vi "Refresh All Pages.vi"() -> ()   [LabVIEW 2014]
uses:
  <vilib>/Platform/browser.llb/Open URL in Default Browser (string).vi
panel:
  in  "Wiki Help Base URL":string="https://www.labviewmakerhub.com/doku.php?id=learn:libraries:linx:reference:labview:"
  out "Array":string[](array[string])=["\\analog-read-1-chan.txt", "\\analog-read-n-chans.txt", "\\analog-set-reference-voltage.txt", "\\analog-write-1-chan.txt", "\\analog-write-n-chans.txt", "\\check-channel.txt", "\\close.txt", "\\custom-command.txt", "\\digital-close.txt", "\\digital-read-1-chan.txt", "\\digital-read-n-chans.txt", "\\digital-read-pulse-width.txt", "\\digital-write-1-chan.txt", "\\digital-write-n-chans.txt", "\\digital-write-square-wave.txt", "\\get-device-user-id.txt", "\\i2c-close.txt", "\\i2c-open.txt", "\\i2c-read.txt", "\\i2c-write.txt", "\\initialize.txt", "\\open-local.txt", "\\open-serial.txt", "\\open-tcp.txt", "\\photocell.txt", "\\pwm-set-duty-cycle-1-chan.txt", "\\pwm-set-duty-cycle-n-chans.txt", "\\rgb-led.txt", "\\set-device-user-id.txt", "\\seven-segment-display.txt", "\\spi-configure.txt", "\\spi-open.txt", "\\spi-write-read-1-frame.txt", "\\spi-write-read-n-frames.txt", "\\thermistor.txt", "\\thumbstick.txt", "\\uart-close.txt", "\\uart-get-bytes-available.txt", "\\uart-open.txt", "\\uart-read-byte-array.txt", "\\uart-read-string.txt", "\\uart-set-baud-rate.txt", "\\uart-write-byte-array.txt", "\\uart-write-string.txt", "\\ad9850\\open.txt", "\\ad9850\\set-frequency-and-phase.txt", "\\adxl345\\close.txt", "\\adxl345\\open.txt", "\\adxl345\\read.txt", "\\blinkm\\go-to-rgb-color-now.txt", "\\blinkm\\open.txt", "\\ds1307\\open.txt", "\\ds1307\\read.txt", "\\ds1307\\write.txt", "\\hitechnic\\accelerometer\\close.txt", "\\hitechnic\\accelerometer\\open.txt", "\\hitechnic\\accelerometer\\read.txt", "\\ltc2631\\open.txt", "\\ltc2631\\write.txt", "\\mma8451\\close.txt", "\\mma8451\\open.txt", "\\mma8451\\read.txt", "\\mma8451\\who-am-i.txt", "\\mma8452\\close.txt", "\\mma8452\\open.txt", "\\mma8452\\read.txt", "\\mpu60x0\\close.txt", "\\mpu60x0\\open.txt", "\\mpu60x0\\read.txt", "\\mpu60x0\\set-clock-source.txt", "\\mpu60x0\\set-fullscale-accel-range.txt", "\\mpu60x0\\set-fullscale-gyro-range.txt", "\\mpu60x0\\set-sleep-enabled.txt", "\\pmodacl\\close.txt", "\\pmodacl\\open.txt", "\\pmodacl\\read.txt", "\\pmodals\\open.txt", "\\pmodals\\read.txt", "\\pmodcmps\\close.txt", "\\pmodcmps\\open.txt", "\\pmodcmps\\read.txt", "\\pmodgyro\\close.txt", "\\pmodgyro\\open.txt", "\\pmodgyro\\read.txt", "\\pmodmic3\\open.txt", "\\pmodmic3\\read.txt", "\\pmodtc1\\open.txt", "\\pmodtc1\\read.txt", "\\servo\\servo-close-n-channels.txt", "\\servo\\servo-close-one-channel.txt", "\\servo\\servo-open-n-channels.txt", "\\servo\\servo-open-one-channel.txt", "\\servo\\servo-set-pulse-width-n-channels.txt", "\\servo\\servo-set-pulse-width-one-channel.txt", "\\ssd1306\\2d-bool-array-to-image-data-helper.txt", "\\ssd1306\\channels-fgv.txt", "\\ssd1306\\digilent-basic-io-shield---oled-config.txt", "\\ssd1306\\digilent-basic-io-shield---oled-draw-bool-array.txt", "\\ssd1306\\enable-charge-pump.txt", "\\ssd1306\\open.txt", "\\ssd1306\\png-to-bool-array.txt", "\\ssd1306\\set-column-address-range.txt", "\\ssd1306\\set-com-hw-config.txt", "\\ssd1306\\set-com-output-scan-direction.txt", "\\ssd1306\\set-display-on-off.txt", "\\ssd1306\\set-page.txt", "\\ssd1306\\set-segment-remap.txt", "\\ssd1306\\write-data.txt", "\\tcn75a\\open.txt", "\\tcn75a\\read.txt", "\\tmp3x\\tmp35.txt", "\\tmp3x\\tmp36.txt", "\\tmp3x\\tmp37.txt", "\\ultrasonic\\gh-311.txt", "\\ultrasonic\\hc-sr04.txt", "\\ultrasonic\\ping.txt", "\\ultrasonic\\read.txt", "\\ws2812\\close.txt", "\\ws2812\\open.txt", "\\ws2812\\refresh.txt", "\\ws2812\\write-n-leds.txt", "\\ws2812\\write-one-led.txt"]
  in  "File Path Control":path=path "C:/Users/samkristoff/Desktop/Online Help/output/data/pages"
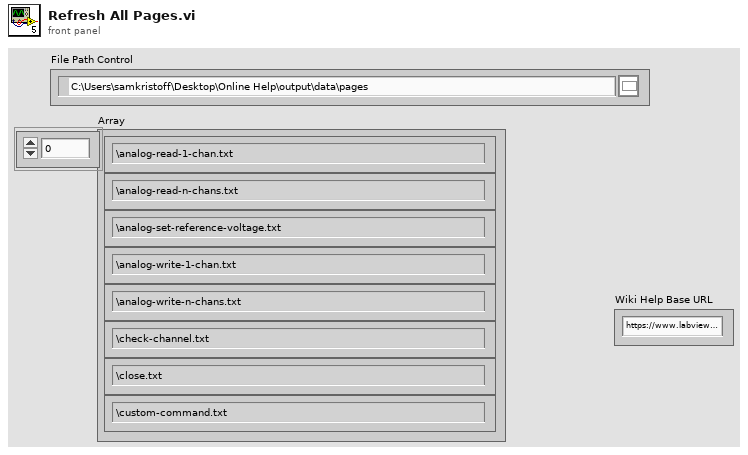
[diagram p1: front panel]
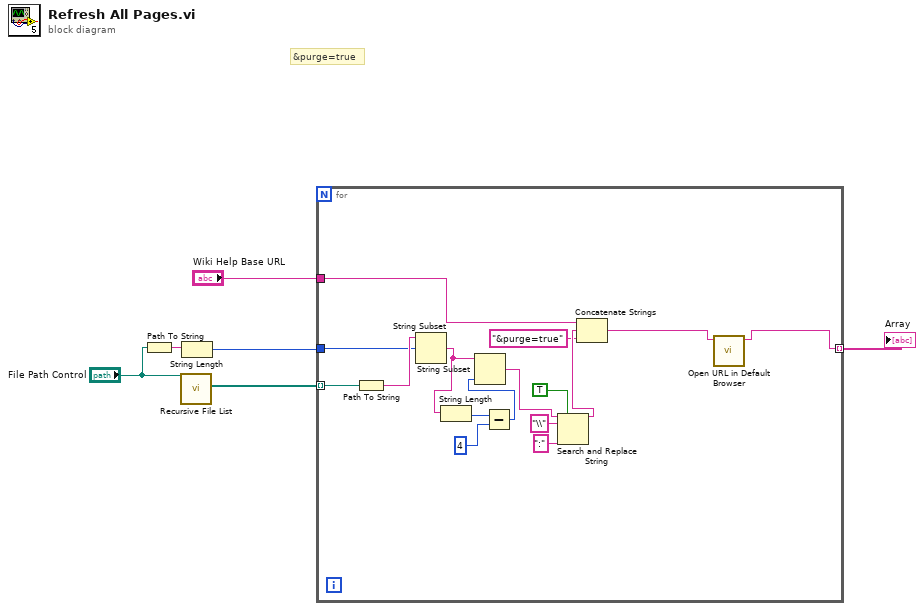
[diagram p0: block diagram]
diagram:
  # "&purge=true"
  n1 = Path To String(path="File Path Control") -> (string=w5:string)
  n2 = call <vilib>:"Recursive File List.vi"("Folder Path"="File Path Control") -> ("All Files in Dir"=w6:path[])  [unwired: 6 in, 4 out]
  n3 = String Length(string=w5) -> (length=w3:i32)
  n4 = for {
    tunnel: w6 -> [w22] mode=indexing
    tunnel: w3 -> [w20]
    tunnel: [w7] -> w2 mode=indexing
    tunnel: "Wiki Help Base URL" -> [w19]
    n5 = Path To String(path=w22) -> (string=w21:string)
    n6 = String Subset(string=w21, offset (0)=w20) -> (substring=w13:string)  [unwired: 1 in]
    n7 = String Length(string=w13) -> (length=w12:i32)
    n8 = Subtract(x=w12, y=4) -> (x-y=w10:i32)
    n9 = String Subset(string=w13, length (rest)=w10) -> (substring=w14:string)  [unwired: 1 in]
    n10 = Search and Replace String(replace all?=TRUE ("replace all? (F)"), input string=w14, search string="\\", replace string=":" ("replace string (\"\")")) -> (result string=w15:string)  [unwired: 4 in, 3 out]
    n11 = Concatenate Strings(w19, w15, "&purge=true" ("string")) -> (w8:string)
    n12 = call-poly <vilib>:"Open URL in Default Browser.vi"("URL"=w8) -> ("URL out"=w7:string)  [unwired: 5 in, 1 out]
  }
  "Array" <- w2
